vi "Add to Flushed Data Size.vi"(10 "TDMS Data Written":dbl[][](array[numeric]), 11 "Flushed Data Size In":u32) -> (3 "Flushed Data Size Out":u32)   [LabVIEW 2027, in "Embedded Data Logger Engine.lvlib"]
uses:
  Embedded Data Logger Engine.lvlib
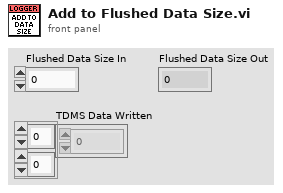
[diagram p1: front panel]
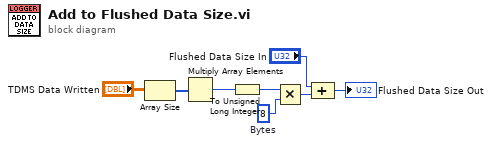
[diagram p0: block diagram]
diagram:
  w3 = u32 8  # Bytes
  n1 = Array Size(array="TDMS Data Written") -> (size(s)=w2:i32[])
  n2 = Multiply Array Elements(1:w2) -> (0:w5:i32)
  n3 = To Unsigned Long Integer(number=w5) -> (unsigned 32bit integer=w1:u32)
  n4 = Multiply(x=w1, y=w3) -> (x*y=w6:u32)
  n5 = Compound Arithmetic op=ADD("Flushed Data Size In", w6) -> (→"Flushed Data Size Out":u32)
